vi "Proceed next Image.vi"(8 "error in (no error)":errorcluster, 11 "Launch File Viewer in":refnum<class "HIJ Vision File Viewer App.lvclass">) -> (0 "error out":errorcluster, 3 "Launch File Viewer out":refnum<class "HIJ Vision File Viewer App.lvclass">)   [LabVIEW 2014, in "HIJ Vision File Viewer App.lvlib" / "HIJ Vision File Viewer App.lvclass"]
uses:
  HIJ Vision File Viewer App.lvclass
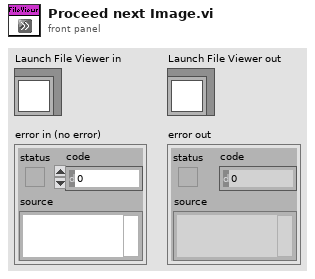
[diagram p1: front panel]
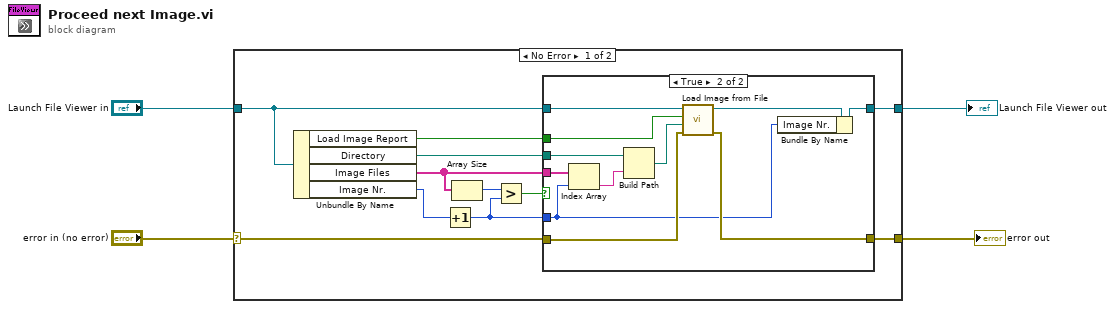
[diagram p0: block diagram]
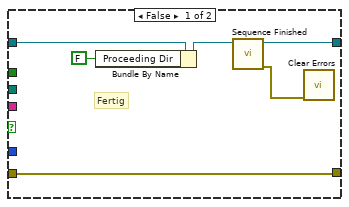
[diagram p2: hidden frame]
diagram:
  n1 = case shown="No Error" "error in (no error)" {
    selector: "error in (no error)" -> [w6 w34]
    tunnel: [w5 w34] -> w2
    tunnel: [w14 w33] -> w1
    tunnel: "Launch File Viewer in" -> [w15 w33]
    frame No Error {
      n2 = Unbundle By Name(w15) -> ("Load Image Report"=w11:bool, "Directory"=w12:path, "Image Files"=w10:string[], "Image Nr."=w13:i32)
      n3 = Increment(x=w13) -> (x+1=w8:i32)
      n4 = Array Size(array=w10) -> (size(s)=w9:i32)
      n5 = Greater?(x=w9, y=w8) -> (0:w7:bool)
      n6 = case shown="True" w7 {
        tunnel: w15 -> [w21 w32]
        tunnel: [w17 w25] -> w14
        tunnel: w8 -> [_ w22]
        tunnel: w10 -> [_ w30]
        tunnel: w12 -> [_ w28]
        tunnel: w11 -> [_ w26]
        tunnel: w6 -> [w19 w24]
        tunnel: [w19 w23] -> w5
        frame False {
          # "Fertig"
          n7 = Bundle By Name(cluster=w21, "Proceeding Dir"=FALSE) -> (w18:refnum<class "HIJ Vision File Viewer App.lvclass">)
          n8 = call-dynamic "Sequence Finished.vi"("HIJ Vision Application in"=w18) -> ("error out"=w16:errorcluster, "HIJ Vision Application out"=w17:refnum<class "HIJ Vision File Viewer App.lvclass">)  [unwired: 9 in]
          n9 = call <vilib>:"Clear Errors.vi"("error in (no error)"=w16) -> ()  [unwired: 5 in, 2 out]
        }
        frame True {
          n10 = Index Array(array=w30, index=w22) -> (element=w29:string)
          n11 = Build Path(base path=w28, name or relative path=w29) -> (appended path=w27:path)
          n12 = call-dynamic "Load Image from File.vi"("error in (no error)"=w24, "Image"=w27, "Load Report"=w26, "Launch File Viewer in"=w32) -> ("error out"=w23:errorcluster, "Launch File Viewer out"=w31:refnum<class "HIJ Vision File Viewer App.lvclass">)  [unwired: 6 in]
          n13 = Bundle By Name(cluster=w31, "Image Nr."=w22) -> (w25:refnum<class "HIJ Vision File Viewer App.lvclass">)
        }
      }
    }
    frame Error {
    }
  }
  "error out" <- w2
  "Launch File Viewer out" <- w1
